vi "Stop Collect.vi"(8 "error in (no error)":errorcluster, 10 "dummy":bool) -> (0 "error out":errorcluster, 1 "timed out?":bool, 2 "Reply Payload":T1)   [LabVIEW 2015, in "Collect Data Mgr.lvlib"]
doc: "_____\nCreated using Delacor QMH Event Scripter 2.1.0.3."
uses:
  Collect Data Mgr.lvlib
  Stop Collect (Reply Payload)--cluster.ctl
  Stop Collect Argument--cluster.ctl
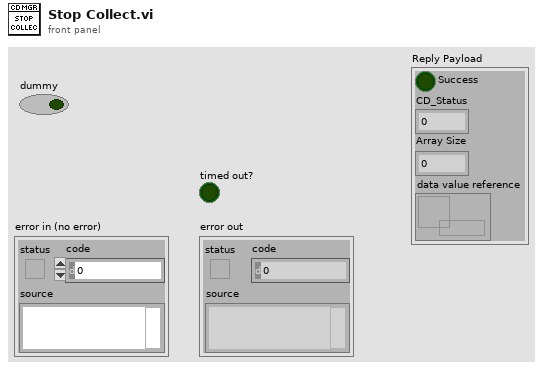
[diagram p1: front panel]
types:
  T1 = typedef "Collect Data Mgr.lvlib/Stop Collect (Reply Payload)--cluster.ctl" = cluster{"Success":bool, "CD_Status":i32, "Array Size":u32, "data value reference":refnum<data-value>}
  T2 = typedef "Collect Data Mgr.lvlib/Stop Collect Argument--cluster.ctl" = cluster{"dummy":bool, "Wait Notifier":refnum<notifier>}
  T3 = typedef "Collect Data Mgr.lvlib/Request Events--cluster.ctl" = cluster{"Stop Module":refnum<user-event>, "Show Panel":refnum<user-event>, "Hide Panel":refnum<user-event>, "Get Module Execution Status":refnum<user-event>, "Show Diagram":refnum<user-event>, "Start Collect":refnum<user-event>, "Stop Collect":refnum<user-event>}
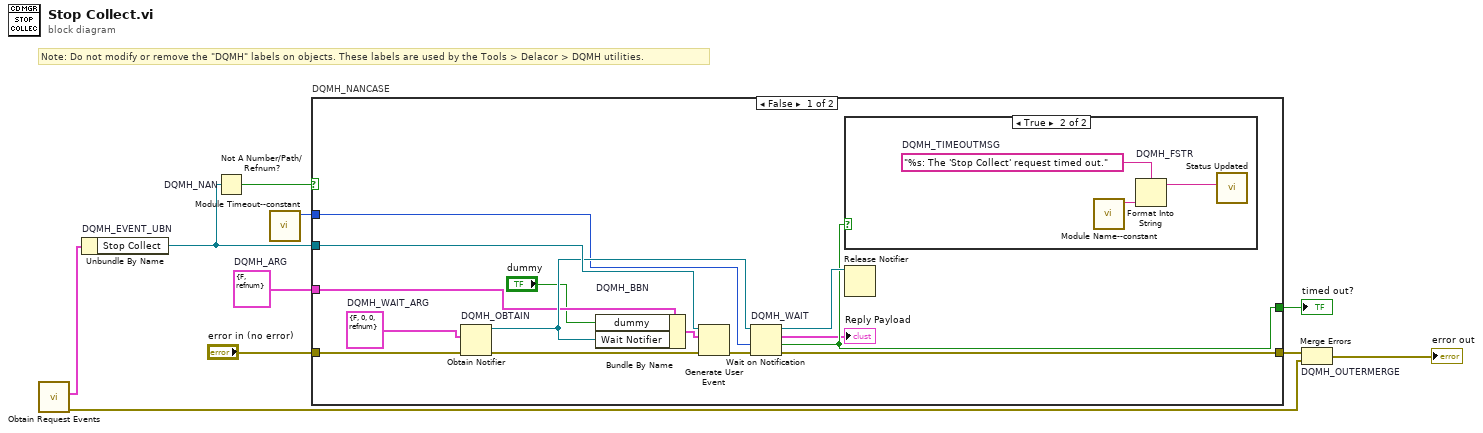
[diagram p0: block diagram]
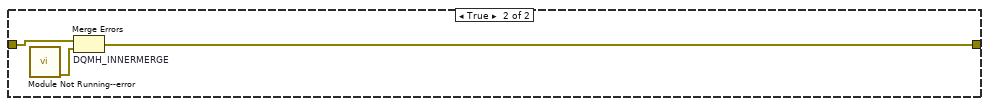
[diagram p3: hidden frame]
diagram:
  w4 = T2 {"dummy"=FALSE, "Wait Notifier"=refnum}  # DQMH_ARG
  # "Note: Do not modify or remove the \"DQMH\" labels on objects. These labels are used by the Tools > Delacor > DQMH utilities."
  n1 = call "Obtain Request Events.vi"() -> ("error out"=w2:errorcluster, "Probe Mgr Request Events"=w1:T3)  [unwired: 10 in]
  n2 = Unbundle By Name "DQMH_EVENT_UBN"(w1) -> ("Stop Collect"=w8:refnum<user-event>)
  n3 = Not A Number/Path/Refnum? "DQMH_NAN"(number/path/refnum=w8) -> (NaN/Path/Refnum?=w7:bool)
  n4 = call "Module Timeout--constant.vi"() -> ("Module Timeout"=w3:i32)  [unwired: 11 in]
  n5 = case "DQMH_NANCASE" shown="False" w7 {
    tunnel: "error in (no error)" -> [w24 w30]
    tunnel: w8 -> [w22 _]
    tunnel: [w18 w29] -> w5
    tunnel: [w15 _] -> w6
    tunnel: w4 -> [w14 _]
    tunnel: w3 -> [w12 _]
    frame False {
      w19 = T1 {"Success"=FALSE, "CD_Status"=0, "Array Size"=0, "data value reference"=refnum}  # DQMH_WAIT_ARG
      n6 = Obtain Notifier "DQMH_OBTAIN"(notification data type=w19, error in (no error)=w24) -> (notifier out=w17:refnum<notifier>, error out=w20:errorcluster)  [unwired: 2 in, 1 out]
      n7 = Bundle By Name "DQMH_BBN"(cluster=w14, "dummy"="dummy", "Wait Notifier"=w17) -> (w21:T2)
      n8 = Generate User Event(user event=w22, event data cluster=w21, error in=w20) -> (error out=w23:errorcluster)  [unwired: 1 in, 1 out]
      n9 = Wait on Notification "DQMH_WAIT"(notifier=w17, timeout in ms (-1)=w12, error in (no error)=w23) -> (notifier out=w16:refnum<notifier>, notification=→"Reply Payload":T1, timed out?=w15:bool, error out=w18:errorcluster)  [unwired: 1 in]
      n10 = case shown="True" w15 {
        frame False {
        }
        frame True {
          w27 = "%s: The 'Stop Collect' request timed out."  # DQMH_TIMEOUTMSG
          n11 = call "Module Name--constant.vi"() -> ("Module Name"=w26:string)  [unwired: 11 in]
          n12 = Format Into String "DQMH_FSTR"(format string=w27, w26) -> (resulting string=w25:string)  [unwired: 2 in, 1 out]
          n13 = call "Status Updated.vi"("Status"=w25) -> ()  [unwired: 10 in, 1 out]
        }
      }
      n14 = Release Notifier(notifier=w16) -> ()  [unwired: 2 in, 3 out]
    }
    frame True {
      n15 = call "Module Not Running--error.vi"() -> ("error out"=w28:errorcluster)  [unwired: 11 in]
      n16 = Merge Errors "DQMH_INNERMERGE"(w30, w28) -> (w29:errorcluster)
    }
  }
  "timed out?" <- w6
  n17 = Merge Errors "DQMH_OUTERMERGE"(w5, w2) -> (→"error out":errorcluster)
